vi "Format Timeleft String.vi"(11 "second":dbl) -> (3 "Elapsed Time":string)   [LabVIEW 2020, in "CSM-ScheduledCmdWindow.lvlib"]
uses:
  CSM-ScheduledCmdWindow.lvlib
  <userlib>/_NEVSTOP/Communicable State Machine(CSM)/Communicable State Machine.lvlib
panel:
  out "appended array":i32[](array[numeric])
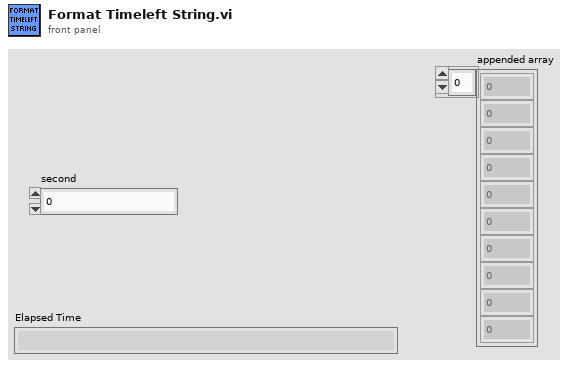
[diagram p1: front panel]
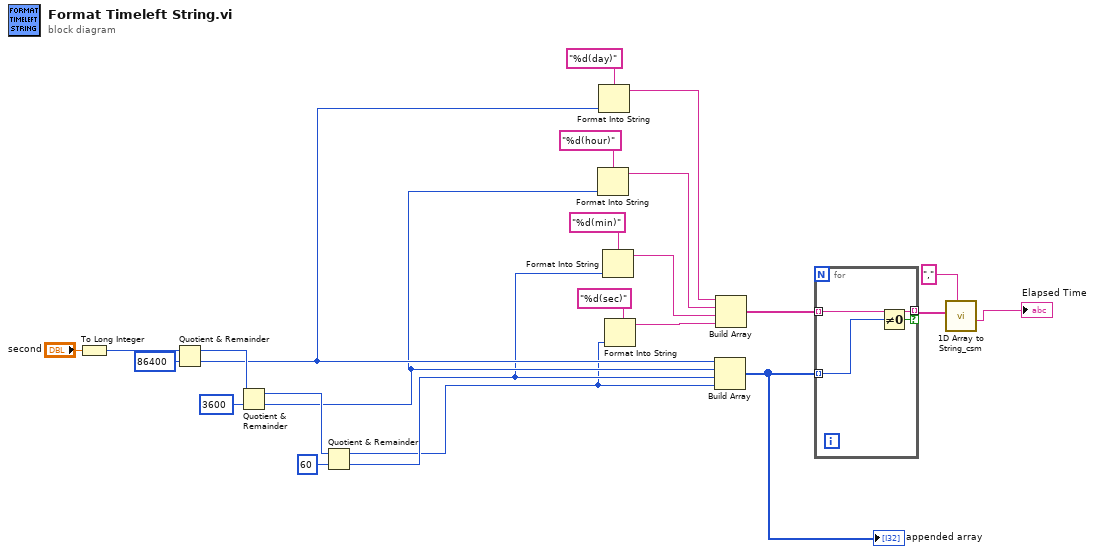
[diagram p0: block diagram]
diagram:
  n1 = To Long Integer(number="second") -> (32bit integer=w20:i32)
  n2 = Quotient & Remainder(x=w20, y=86400) -> (x-y*floor(x/y)=w22:i32, floor(x/y)=w17:i32)
  n3 = Quotient & Remainder(x=w22, y=3600) -> (x-y*floor(x/y)=w18:i32, floor(x/y)=w14:i32)
  n4 = Quotient & Remainder(x=w18, y=60) -> (x-y*floor(x/y)=w10:i32, floor(x/y)=w12:i32)
  n5 = Format Into String(format string="%d(hour)", w14) -> (resulting string=w7:string)  [unwired: 2 in, 1 out]
  n6 = Format Into String(format string="%d(day)", w17) -> (resulting string=w6:string)  [unwired: 2 in, 1 out]
  n7 = Format Into String(format string="%d(min)", w12) -> (resulting string=w8:string)  [unwired: 2 in, 1 out]
  n8 = Format Into String(format string="%d(sec)", w10) -> (resulting string=w9:string)  [unwired: 2 in, 1 out]
  n9 = Build Array(w17, w14, w12, w10) -> (w4:i32[])
  "appended array" <- w4
  n10 = Build Array(w6, w7, w8, w9) -> (w5:string[])
  n11 = for {
    tunnel: [w27] -> w3 mode=indexing if=w25
    tunnel: w5 -> [w27] mode=indexing
    tunnel: w4 -> [w26] mode=indexing
    n12 = Not Equal To 0?(x=w26) -> (x != 0?=w25:bool)
  }
  n13 = call <userlib>:"1D Array to String_csm.vi"("delimiter (Tab)"=",", "Array of Strings"=w3) -> ("delimited string"=→"Elapsed Time":string)  [unwired: 9 in]
